vi "moving_to_wall.vi"(8 "error in (no error)":errorcluster, 11 "Distance to wall":dbl format="%#_13g") -> (0 "error out":errorcluster)   [LabVIEW 2016]
uses:
  <vilib>/myRIO/Common/Instrument Driver Framework/myRIO v1.0/Encoder/typedefs/Encoder Signal Mode.ctl
  <vilib>/myRIO/Instrument Drivers/Onboard IO/Encoder/typedefs/Encoder Reference.ctl
  <vilib>/myRIO/Common/Instrument Driver Framework/Utilities/typedefs/myRIO Generic Hardware Reference.ctl
  <vilib>/myRIO/Common/Instrument Driver Framework/Utilities/typedefs/Hardware Version Enum.ctl
  <vilib>/myRIO/Common/Instrument Driver Framework/Utilities/typedefs/myRIO v1.0 Reference.ctl
  <vilib>/myRIO/Common/Instrument Driver Framework/Utilities/typedefs/Generic FPGA Reference.ctl
  <vilib>/myRIO/Common/Instrument Driver Framework/myRIO v1.0/Encoder/typedefs/Encoder Channels Enum.ctl
  <vilib>/myRIO/Common/Instrument Driver Framework/myRIO v1.0/Encoder/typedefs/Encoder Configuration v1.0.ctl
  <vilib>/userdefined/High Color/nirio_resource_hc.ctl
  <vilib>/myRIO/Instrument Drivers/Onboard IO/PWM/typedefs/PWM Reference.ctl
  <vilib>/myRIO/Common/Instrument Driver Framework/myRIO v1.0/PWM/typedefs/PWM Channels Enum.ctl
  <vilib>/myRIO/Instrument Drivers/Onboard IO/PWM/typedefs/PWM Configuration.ctl
  <vilib>/myRIO/Instrument Drivers/Onboard IO/DIO/typedefs/DIO Reference.ctl
  <vilib>/myRIO/Common/Instrument Driver Framework/myRIO v1.0/DIO/typedefs/DIO Channels List.ctl
  <vilib>/myRIO/Common/Instrument Driver Framework/myRIO v1.0/DIO/typedefs/DIO Channels Enum.ctl
  <vilib>/myRIO/Instrument Drivers/Onboard IO/AI/typedefs/AI Reference.ctl
  <vilib>/myRIO/Common/Instrument Driver Framework/myRIO v1.0/AI/typedefs/AI Channels List.ctl
  <vilib>/myRIO/Common/Instrument Driver Framework/myRIO v1.0/AI/typedefs/AI Channels Enum.ctl
  <vilib>/myRIO/Common/Instrument Driver Framework/Utilities/typedefs/Analog Scaling Constants List.ctl
  <vilib>/myRIO/Common/Instrument Driver Framework/Utilities/typedefs/Analog Scaling Constants.ctl
  <vilib>/myRIO/Common/Instrument Driver Framework/Utilities/vis/Is FPGA Ref Available.vi
  <vilib>/myRIO/Common/Instrument Driver Framework/myRIO v1.0/Encoder/vis/myRIO v1.1 Open Encoder.vi
  <vilib>/myRIO/Instrument Drivers/Onboard IO/Encoder/vis/Read.vi
  <vilib>/myRIO/Common/Instrument Driver Framework/myRIO v1.0/PWM/vis/myRIO v1.1 Open PWM.vi
  <vilib>/myRIO/Instrument Drivers/Onboard IO/PWM/vis/Set Duty Cycle and Frequency.vi
  <vilib>/myRIO/Common/Instrument Driver Framework/myRIO v1.0/DIO/vis/myRIO v1.1 Open DIO.vi
  <vilib>/myRIO/Instrument Drivers/Onboard IO/DIO/vis/Write.vi
  <vilib>/myRIO/Common/Instrument Driver Framework/myRIO v1.0/AI/vis/myRIO v1.1 Open AI.vi
  <vilib>/myRIO/Instrument Drivers/Onboard IO/AI/vis/Read.vi
  <vilib>/myRIO/Common/Instrument Driver Framework/Utilities/vis/Validate Channels.vi
  <vilib>/myRIO/Common/Instrument Driver Framework/myRIO v1.0/Encoder/vis/myRIO v1.0 Reserve Encoder.vi
  <vilib>/myRIO/Common/Instrument Driver Framework/myRIO v1.0/PWM/vis/myRIO v1.0 Reserve PWM.vi
  <vilib>/myRIO/Common/Instrument Driver Framework/myRIO v1.0/DIO/vis/myRIO v1.0 Reserve DIO.vi
  <vilib>/myRIO/Common/Instrument Driver Framework/myRIO v1.0/AI/vis/myRIO v1.0 Reserve AI.vi
  <vilib>/myRIO/Common/Instrument Driver Framework/myRIO v1.0/Encoder/vis/myRIO v1.0 Build MUX Configuration Encoder.vi
  <vilib>/myRIO/Common/Instrument Driver Framework/myRIO v1.0/Resource Manager/vis/myRIO v1.0 Reserve Channel List.vi
  <vilib>/myRIO/Common/Instrument Driver Framework/myRIO v1.0/PWM/vis/myRIO v1.0 Build MUX Configuration PWM.vi
  <vilib>/myRIO/Common/Instrument Driver Framework/myRIO v1.0/DIO/vis/myRIO v1.0 Build MUX Configuration DIO.vi
  <vilib>/myRIO/Common/Instrument Driver Framework/myRIO v1.0/AI/vis/myRIO v1.0 Build MUX Configuration AI.vi
  <vilib>/myRIO/Common/Instrument Driver Framework/myRIO v1.0/Resource Manager/vis/myRIO v1.0 Create Configuration List.vi
  <vilib>/myRIO/Common/Instrument Driver Framework/myRIO v1.0/Resource Manager/vis/myRIO v1.0 Reserve Channel.vi
  <vilib>/myRIO/Common/Instrument Driver Framework/myRIO v1.0/Resource Manager/vis/myRIO v1.0 Unreserve Channel.vi
  <vilib>/myRIO/Common/Instrument Driver Framework/myRIO v1.0/Resource Manager/vis/myRIO v1.0 Build Mutex Name.vi
  <vilib>/Utility/VariantDataType/GetNumericInfo.vi
  <vilib>/Utility/error.llb/Error Cluster From Error Code.vi
  <vilib>/myRIO/Common/Instrument Driver Framework/myRIO v1.0/myRIO v1.1 Open.vi
  <vilib>/myRIO/Common/Instrument Driver Framework/myRIO v1.0/AI/vis/myRIO v1.0 Get Scaling Constants AI.vi
  <vilib>/myRIO/Common/Instrument Driver Framework/Utilities/vis/IO Manager.vi
  <vilib>/myRIO/Common/Instrument Driver Framework/Utilities/vis/Configuration Manager.vi
  <vilib>/myRIO/Common/Instrument Driver Framework/myRIO v1.0/myRIO v1.0 Close.vi
  <vilib>/myRIO/Common/Instrument Driver Framework/myRIO v1.0/AI/vis/myRIO v1.0 Read AI.vi
  <vilib>/myRIO/Common/Instrument Driver Framework/myRIO v1.0/Resource Manager/vis/myRIO v1.0 Configure IO.vi
  <vilib>/myRIO/Common/Instrument Driver Framework/myRIO v1.0/Encoder/vis/myRIO v1.0 Configure Encoder.vi
  <vilib>/myRIO/Common/Instrument Driver Framework/myRIO v1.0/Encoder/vis/myRIO v1.0 Read Encoder.vi
  <vilib>/imath/engines/lvmath2/RunTimeEngine/BuiltInFunctions/abs/NIMS_abs(signed).vi
  <instcachedir>/0/NIMS_abs(signed)_C4FCB8E6058B49B797C7C8D53CA5F6EC.lvgen/NIMS_abs(signed)_C4FCB8E6058B49B797C7C8D53CA5F6EC_007.vi
  <vilib>/imath/engines/lvmath2/RunTimeEngine/NodeEndStatement/NIMS_NodeEndStatement_Output.vi
  <instcachedir>/0/NIMS_NodeEndStatement_Output_53EC0D466D134D7ABD903AC30B43404B.lvgen/NIMS_NodeEndStatement_Output_53EC0D466D134D7ABD903AC30B43404B_001.vi
  <vilib>/imath/engines/lvmath2/RunTimeEngine/ErrorHandling/NIMS_Finalize Error.vi
  <vilib>/myRIO/Common/Instrument Driver Framework/myRIO v1.0/PWM/vis/myRIO v1.0 Write PWM.vi
  <vilib>/myRIO/Common/Instrument Driver Framework/myRIO v1.0/DIO/vis/myRIO v1.0 Write DIO.vi
  <vilib>/myRIO/Express VI/Onboard IO/AI/AI Express VI.xnode
  <vilib>/myRIO/Instrument Drivers/Onboard IO/AI/vis/myRIO AI Open.xnode
  <vilib>/myRIO/Express VI/Onboard IO/Encoder/Encoder Express VI.xnode
  <vilib>/myRIO/Instrument Drivers/Onboard IO/Encoder/vis/myRIO Encoder Open.xnode
  <vilib>/myRIO/Common/Instrument Driver Framework/myRIO v1.0/Encoder/typedefs/Encoder Count Direction Enum.ctl
  <vilib>/myRIO/Express VI/Onboard IO/PWM/PWM Express VI.xnode
  <vilib>/myRIO/Instrument Drivers/Onboard IO/PWM/vis/myRIO PWM Open.xnode
  <vilib>/myRIO/Express VI/Onboard IO/DO/DO Express VI.xnode
  <vilib>/myRIO/Instrument Drivers/Onboard IO/DIO/vis/myRIO DIO Open.xnode
  <vilib>/myRIO/Instrument Drivers/Onboard IO/PWM/PWM.lvlib
  <vilib>/myRIO/Instrument Drivers/Onboard IO/Encoder/Encoder.lvlib
  <vilib>/myRIO/Instrument Drivers/Onboard IO/DIO/DIO.lvlib
  <vilib>/ptbypt/NI_PtbyPt.lvlib
  <vilib>/myRIO/Instrument Drivers/Onboard IO/AI/AI.lvlib
panel:
  out "Stop":bool
  out "Range [cm]":dbl(knob) scale=0.0..80.0
  in  "Kscale [cm-V]":dbl=27.5
  in  "Koffset [cm]":dbl
  in  "[ESC]":bool
  in  "PWM  [%]":dbl(slide)=30.0 scale=-100.0..100.0
  out "Counter Right":i32
  out "PWM Right":dbl
  out "PWM Left":dbl
  out "Counter Left":i32
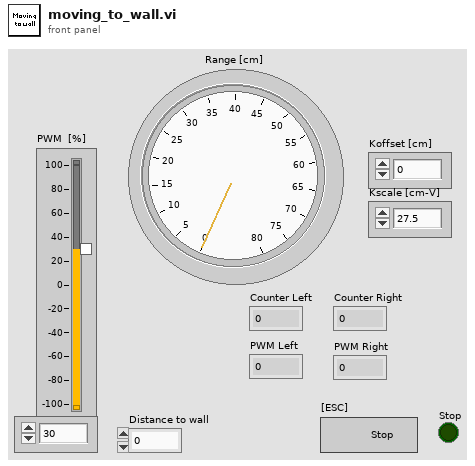
[diagram p1: front panel]
types:
  T1 = typedef "Encoder.lvlib/Encoder Reference.ctl" = cluster{"myRIO Reference":T2, "Encoder Channels Enum":T6}
  T2 = typedef "myRIO Generic Hardware Reference.ctl" = cluster{"myRIO Model":T3, "myRIO Hardware Reference":T4}
  T3 = typedef "Hardware Version Enum.ctl" = enum16{"Unknown", "myRIO-1900", "myRIO-1950", "roboRIO", "NI ELVIS RIO CM"}
  T4 = typedef "myRIO v1.0 Reference.ctl" = cluster{"Generic FPGA Reference":T5, "Allow multiple opens":bool}
  T5 = typedef "Generic FPGA Reference.ctl" = refnum<k20>
  T6 = typedef "Encoder Channels Enum.ctl" = enum16{"Not Connected", "C/ENC0", "C/ENC1", "A/ENC", "B/ENC", "DIO/ENC0", "DIO/ENC1", "DIO/ENC2", "DIO/ENC3", "DIO/ENC4"}
  T7 = typedef "Encoder Signal Mode.ctl" = enum16{"Quadrature phase signal", "Step and direction signal"}
  T8 = typedef "nirio_resource_hc.ctl" = tag
  T9 = typedef "DIO.lvlib/DIO Reference.ctl" = cluster{"myRIO Reference":T2, "DIO Channels List":T10}
  T10 = typedef "DIO Channels List.ctl" = T11[]
  T11 = typedef "DIO Channels Enum.ctl" = enum16{"Not Connected", "C/DIO0", "C/DIO1", "C/DIO2", "C/DIO3", "C/DIO4", "C/DIO5", "C/DIO6", "C/DIO7", "A/DIO0", "A/DIO1", "A/DIO2", "A/DIO3", "A/DIO4", "A/DIO5", "A/DIO6", "A/DIO7", "A/DIO8", "A/DIO9", "A/DIO10", "A/DIO11", "A/DIO12", "A/DIO13", "A/DIO14", "A/DIO15", "B/DIO0", "B/DIO1", "B/DIO2", "B/DIO3", "B/DIO4", "B/DIO5", "B/DIO6", "B/DIO7", "B/DIO8", "B/DIO9", "B/DIO10", "B/DIO11", "B/DIO12", "B/DIO13", "B/DIO14", "B/DIO15", "LED0", "LED1", "LED2", "LED3", "Button0", "DIO/DIO0", "DIO/DIO1", "DIO/DIO2", "DIO/DIO3", "DIO/DIO4", "DIO/DIO5", "DIO/DIO6", "DIO/DIO7", "DIO/DIO8", "DIO/DIO9", "SPI/CS0", "SPI/CS1", "SPI/CS2", "SPI/CS3", "LED RADIO (Green)", "LED RADIO (Red)", "LED COMM (Green)", "LED COMM (Red)", "LED MODE (Green)", "LED MODE (Red)"}
  T12 = typedef "PWM.lvlib/PWM Reference.ctl" = cluster{"myRIO Reference":T2, "PWM Channels Enum":T13, "PWM Configuration":T14}
  T13 = typedef "PWM Channels Enum.ctl" = enum16{"Not Connected", "C/PWM0", "C/PWM1", "A/PWM0", "A/PWM1", "A/PWM2", "B/PWM0", "B/PWM1", "B/PWM2", "PWM/PWM0", "PWM/PWM1", "PWM/PWM2", "PWM/PWM3", "PWM/PWM4", "PWM/PWM5", "PWM/PWM6", "PWM/PWM7", "PWM/PWM8", "PWM/PWM9"}
  T14 = typedef "PWM.lvlib/PWM Configuration.ctl" = cluster{"Frequency":dbl, "Duty Cycle":dbl}
  T15 = typedef "AI.lvlib/AI Reference.ctl" = cluster{"myRIO Reference":T2, "AI Channels List":T16, "AI Scaling Constants List":T18}
  T16 = typedef "AI Channels List.ctl" = T17[]
  T17 = typedef "AI Channels Enum.ctl" = enum16{"Not Connected", "AudioIn/Left", "AudioIn/Right", "C/AI0", "C/AI1", "A/AI0", "A/AI1", "A/AI2", "A/AI3", "B/AI0", "B/AI1", "B/AI2", "B/AI3", "AI/AI0", "AI/AI1", "AI/AI2", "AI/AI3"}
  T18 = typedef "Analog Scaling Constants List.ctl" = T19[]
  T19 = typedef "Analog Scaling Constants.ctl" = cluster{"LSB Weight (Volts)":dbl, "Offset (Volts)":dbl, "Signed?":bool}
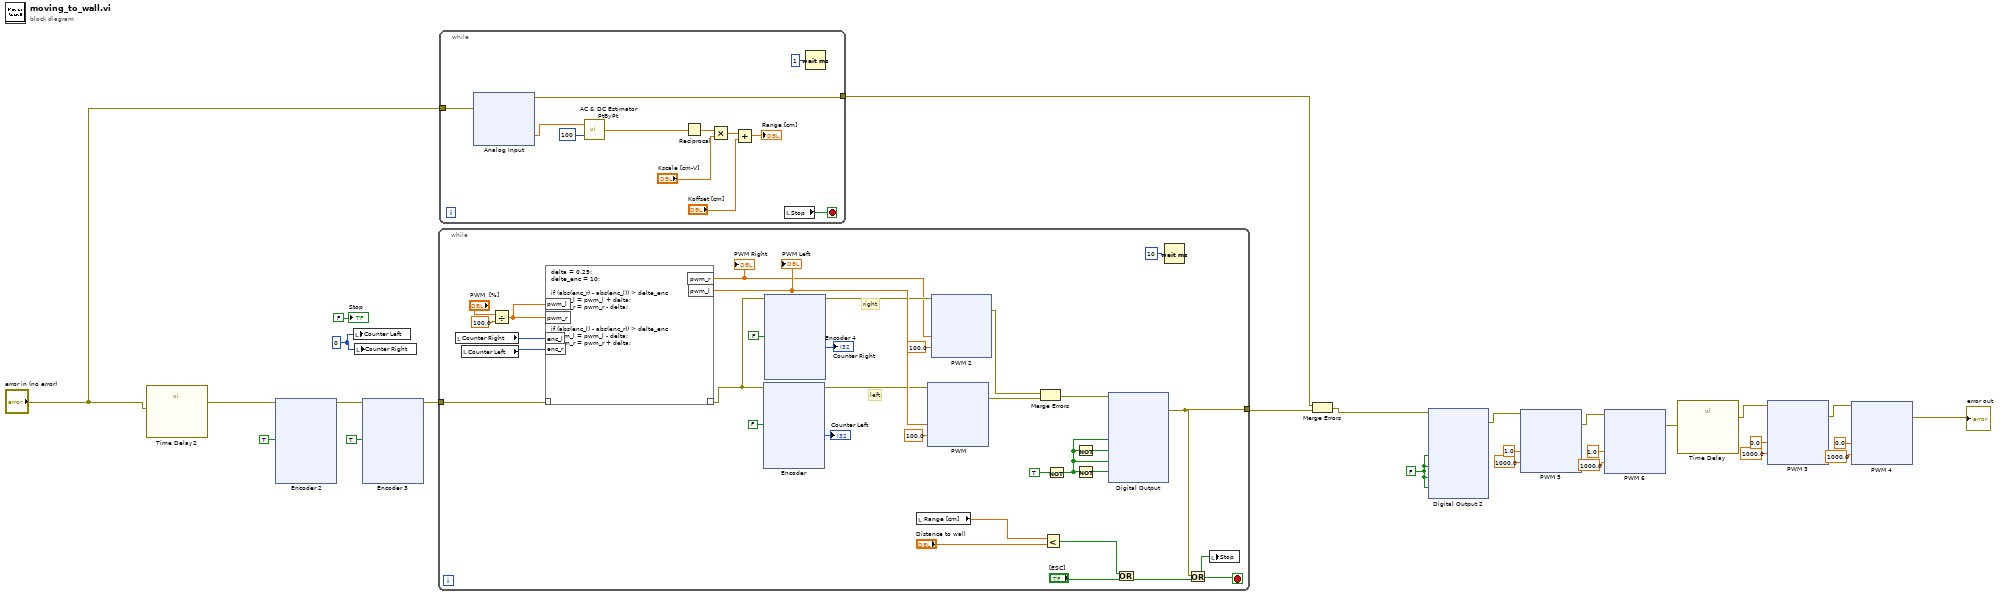
[diagram p0: block diagram]
diagram:
  w15 = FALSE
  w22 = 0
  n1 = call "Time Delay2"("error in (no error)"="error in (no error)") -> ("error out"=w1:errorcluster)  [unwired: 10 in]
  n2 = xnode "Encoder 2"("Reset Counter"=TRUE, "error in (no error)"=w1) -> ("error out"=w24:errorcluster)  [unwired: 3 out]
  n3 = local write "Counter Left"(w22) -> ()
  n4 = local write "Counter Right"(w22) -> ()
  n5 = xnode "Encoder 3"("Reset Counter"=TRUE, "error in (no error)"=w24) -> ("error out"=w23:errorcluster)  [unwired: 3 out]
  n6 = while {
    tunnel: w23 -> [w54]
    tunnel: [w33] -> w5
    stop <- w32 stop-if-true
    # "left"
    # "right"
    n7 = local read "Counter Right"() -> (w45:i32)
    n8 = local read "Counter Left"() -> (w39:i32)
    n9 = Divide(x="PWM  [%]", y=100.0) -> (x/y=w55:dbl)
    n10 = mathscript code="delta = 0.25;\ndelte_enc = 10;\n\nif (abs(enc_r) - abs(enc_l)) > delte_enc\n  pwm_l = pwm_l + delta;\n  pwm_r = pwm_r - delta;\nend\n\nif (abs(enc_l) - abs(enc_r)) > delte_enc\n  pwm_l = pwm_l - delta;\n  pwm_r = pwm_r + delta;\nend"("??"=w54, "pwm_l"=w55, "pwm_r"=w55, "enc_l"=w45, "enc_r"=w39) -> ("??"=w43:errorcluster, "pwm_l"=w50:dbl, "pwm_r"=w35:dbl)
    "PWM Right" <- w35
    "PWM Left" <- w50
    n11 = xnode "Encoder"("Reset Counter"=FALSE, "error in (no error)"=w43) -> ("Counter Value"=→"Counter Left":i32, "error out"=w42:errorcluster)  [unwired: 2 out]
    n12 = xnode "Encoder 4"("Reset Counter"=FALSE, "error in (no error)"=w43) -> ("Counter Value"=→"Counter Right":i32, "error out"=w41:errorcluster)  [unwired: 2 out]
    n13 = local read "Range [cm]"() -> (w31:dbl)
    n14 = xnode "PWM"("Duty Cycle"=w50, "Frequency [Hz]"=100.0, "error in (no error)"=w42) -> ("error out"=w52:errorcluster)
    n15 = xnode "PWM 2"("Duty Cycle"=w35, "Frequency [Hz]"=100.0, "error in (no error)"=w41) -> ("error out"=w53:errorcluster)
    n16 = Merge Errors(w53, w52) -> (w51:errorcluster)
    n17 = Less?(x=w31, y="Distance to wall") -> (x < y?=w27:bool)
    n18 = Not(x=TRUE) -> (.not. x?=w36:bool)
    n19 = Not(x=w36) -> (.not. x?=w38:bool)
    n20 = Not(x=w36) -> (.not. x?=w37:bool)
    n21 = xnode "Digital Output"("M0 Enable (A/DIO5 (Pin 21))"=w36, "M0 Reverse (A/DIO6 (Pin 23))"=w38, "M1 Enable (A/DIO7 (Pin 25))"=w36, "M1 Reverse (A/DIO13 (Pin 26))"=w37, "error in (no error)"=w51) -> ("error out"=w33:errorcluster)
    n22 = Or(x=w27, y="[ESC]") -> (x .or. y?=w29:bool)
    n23 = Wait (ms)(milliseconds to wait=u32 10) -> ()  [unwired: 1 out]
    n24 = Or(x=w33, y=w29) -> (x .or. y?=w32:bool)
    n25 = local write "Stop"(w32) -> ()
  }
  n26 = while {
    tunnel: [w362] -> w4
    tunnel: "error in (no error)" -> [w357]
    stop <- w359 stop-if-true
    n27 = xnode "Analog Input"("error in (no error)"=w357) -> ("A/AI0 (Pin 3)"=w360:dbl, "error out"=w362:errorcluster)
    n28 = call <vilib>:"AC & DC Estimator PtByPt.vi"("signal"=w360, "sample length"=100) -> ("DC estimate (V)"=w366:dbl)  [unwired: 1 in, 2 out]
    n29 = Reciprocal(x=w366) -> (1/x=w368:dbl)
    n30 = Multiply(x=w368, y="Kscale [cm-V]") -> (x*y=w363:dbl)
    n31 = Add(x=w363, y="Koffset [cm]") -> (x+y=→"Range [cm]":dbl)
    n32 = local read "Stop"() -> (w359:bool)
    n33 = Wait (ms)(milliseconds to wait=u32 1) -> ()  [unwired: 1 out]
  }
  n34 = Merge Errors(w4, w5) -> (w3:errorcluster)
  n35 = xnode "Digital Output 2"("M0 Enable (A/DIO5 (Pin 21))"=w15, "M0 Reverse (A/DIO6 (Pin 23))"=w15, "M1 Enable (A/DIO7 (Pin 25))"=w15, "M1 Reverse (A/DIO13 (Pin 26))"=w15, "error in (no error)"=w3) -> ("error out"=w10:errorcluster)
  n36 = xnode "PWM 5"("Duty Cycle"=1.0, "Frequency [Hz]"=1000.0, "error in (no error)"=w10) -> ("error out"=w9:errorcluster)
  n37 = xnode "PWM 6"("Duty Cycle"=1.0, "Frequency [Hz]"=1000.0, "error in (no error)"=w9) -> ("error out"=w8:errorcluster)
  n38 = call "Time Delay"("error in (no error)"=w8) -> ("error out"=w17:errorcluster)  [unwired: 10 in]
  n39 = xnode "PWM 3"("Duty Cycle"=0.0, "Frequency [Hz]"=1000.0, "error in (no error)"=w17) -> ("error out"=w16:errorcluster)
  n40 = xnode "PWM 4"("Duty Cycle"=0.0, "Frequency [Hz]"=1000.0, "error in (no error)"=w16) -> ("error out"=→"error out":errorcluster)
  "Stop" <- FALSE ("Stop")
